vi "line_profile.vi"(0 "Motor COM in":refnum<visa-resource-name>, 1 "Motor error in":errorcluster caption="error out", 2 "Y轴":bool=TRUE, 4 "Keithley COM In":refnum<visa-resource-name>, 5 "Keithley Error In":errorcluster caption="error out", 7 "步长":dbl format="%#_13g", 9 "距离":dbl format="%#_13g", 10 "反向":bool=TRUE) -> (3 "当前位置":dbl format="%#_13g", 12 "XY图":cluster{"X":dbl, "Y":dbl}[](graph), 13 "电流数组":dbl[](array[numeric]), 14 "Motor COM out":refnum<visa-resource-name>, 15 "Motor error out":errorcluster caption="error out", 17 "位移数组":dbl[](array[numeric]), 18 "Keithley COM out":refnum<visa-resource-name>, 19 "Keithley Error out":errorcluster caption="error out")   [LabVIEW 2018]
uses:
  location_x.vi
  location_y.vi
  <instrlib>/Keithley 648X Series/Keithley 648X Series.lvlib
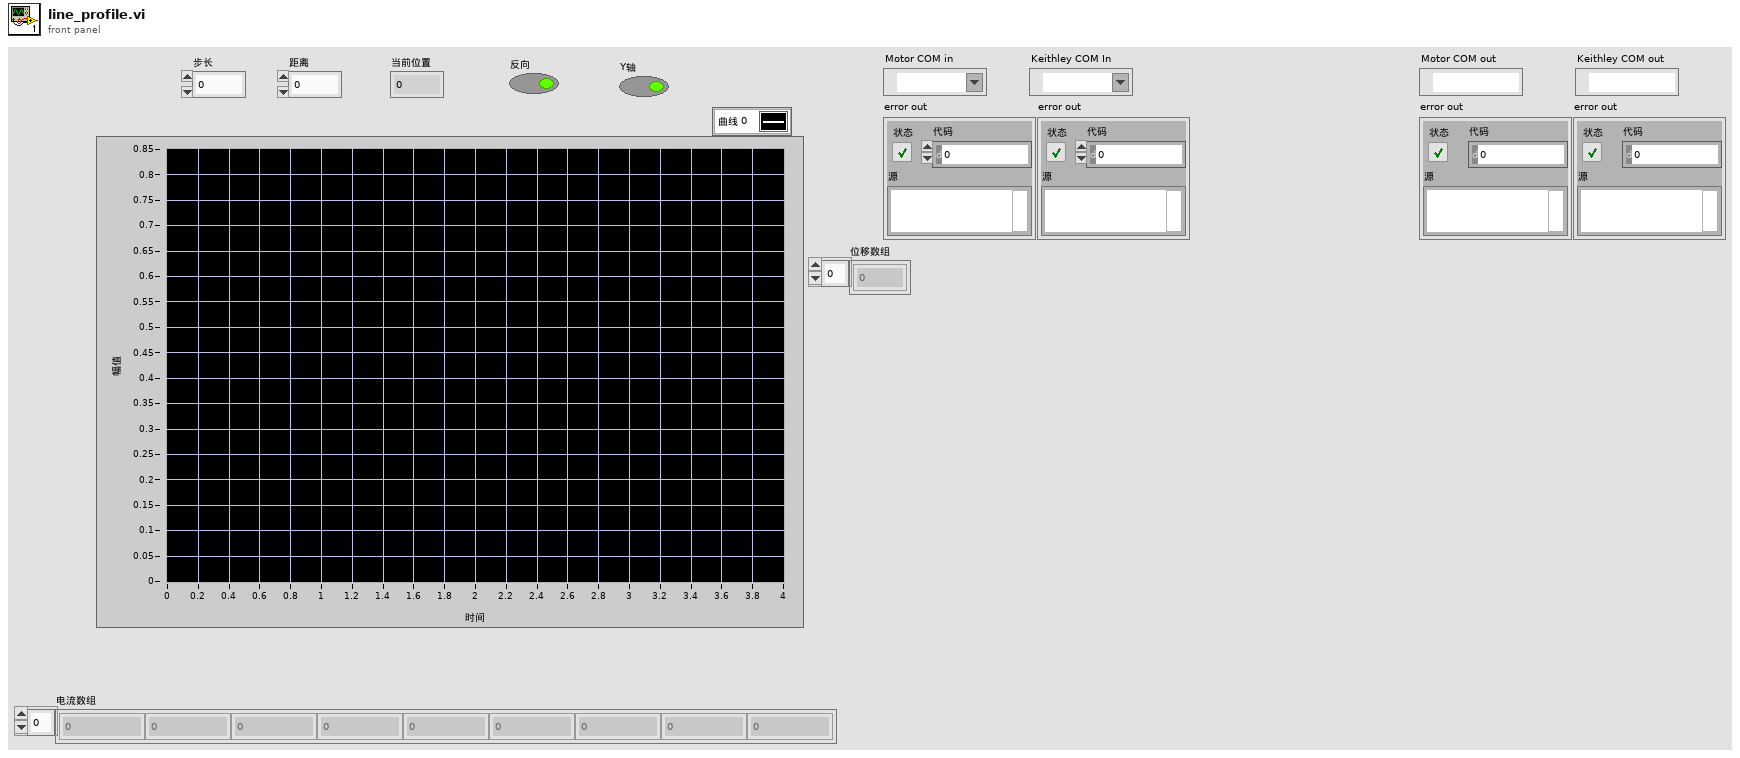
[diagram p1: front panel]
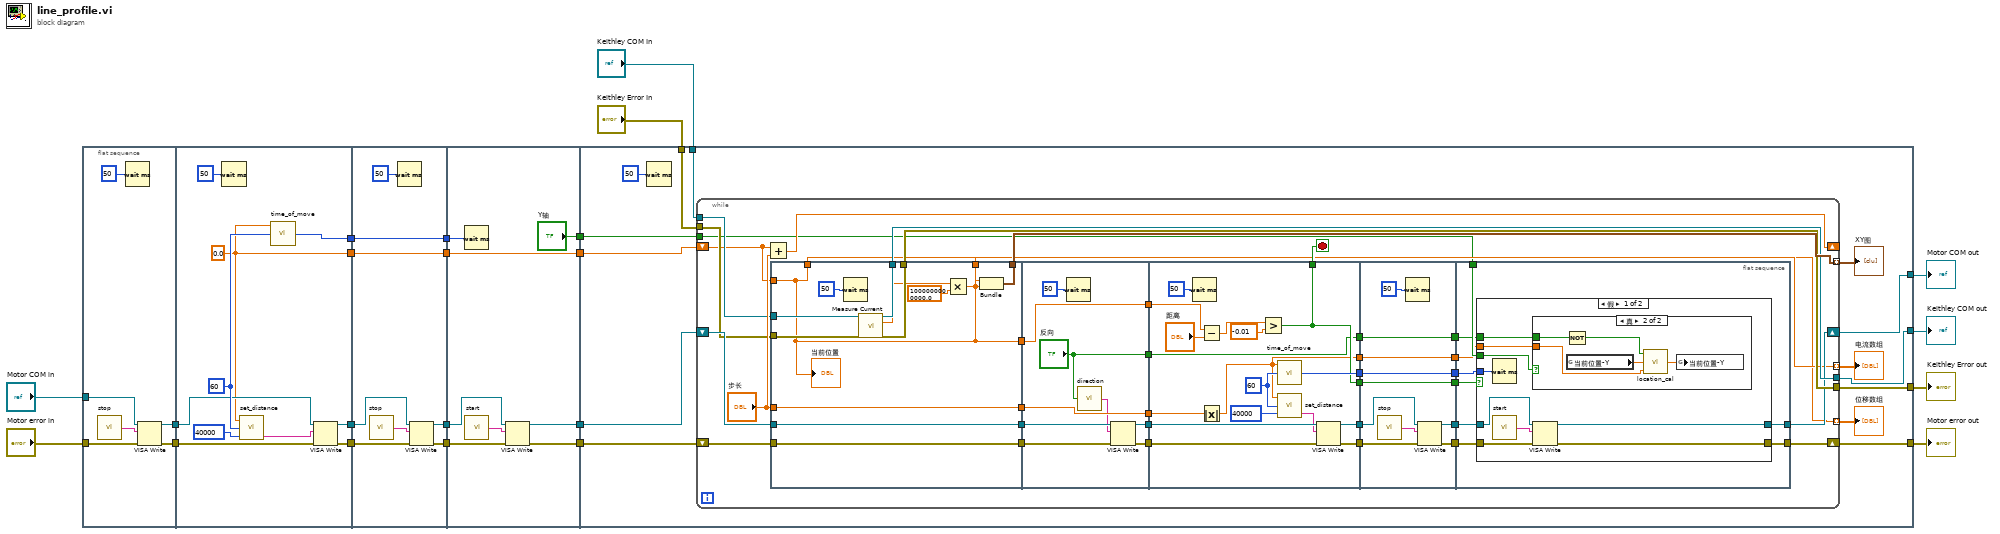
[diagram p0: block diagram]
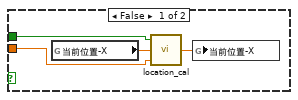
[diagram p2: hidden frame]
diagram:
  n1 = flat-sequence {
    tunnel: "Motor COM in" -> [w28]
    tunnel: "Motor error in" -> [w27]
    tunnel: [w24] -> w22
    tunnel: [w23] -> w21
    tunnel: [w38] -> w20
    tunnel: [w37] -> w19
    tunnel: [w29] -> w18
    tunnel: [w32] -> w17
    tunnel: w22 -> [w31]
    tunnel: w21 -> [w30]
    tunnel: w20 -> [w44]
    tunnel: w19 -> [w46]
    tunnel: [w43] -> w16
    tunnel: [w45] -> w15
    tunnel: [w39] -> w14
    tunnel: w18 -> [w39]
    tunnel: [w40] -> w13
    tunnel: w17 -> [w40]
    tunnel: w16 -> [w52]
    tunnel: w15 -> [w54]
    tunnel: [w51] -> w12
    tunnel: [w53] -> w11
    tunnel: [w49] -> w10
    tunnel: w14 -> [w49]
    tunnel: w13 -> [w48]
    tunnel: ["Y轴"] -> w1
    tunnel: w12 -> [w66]
    tunnel: w11 -> [w68]
    tunnel: w10 -> [w64]
    tunnel: [w65] -> w4
    tunnel: [w67] -> w5
    tunnel: [w59] -> w3
    tunnel: [w58] -> w2
    tunnel: "Keithley Error In" -> [w61]
    tunnel: "Keithley COM In" -> [w60]
    tunnel: w1 -> [w55]
    frame #0 {
      n2 = call "stop.vi"() -> ("指令"=w25:string)
      n3 = Wait (ms)(milliseconds to wait=u32 50 ("毫秒计时值")) -> ()  [unwired: 1 out]
      n4 = VISA Write(VISA resource name=w28, write buffer=w25, error in (no error)=w27) -> (VISA resource name out=w24:refnum<visa-resource-name>, error out=w23:errorcluster)  [unwired: 1 out]
    }
    frame #1 {
      w29 = 0.0
      w33 = i16 60 ("速度(r/min)")
      n5 = Wait (ms)(milliseconds to wait=u32 50 ("毫秒计时值")) -> ()  [unwired: 1 out]
      n6 = call "set_distance.vi"("细分"=40000, "速度(r/min)"=w33, "移动距离(mm)"=w29) -> ("指令"=w35:string)  [unwired: 2 out]
      n7 = call "time_of_move.vi"("转速"=w33, "移动距离"=w29) -> ("所需时间"=w32:i32)  [unwired: 1 in]
      n8 = VISA Write(VISA resource name=w31, write buffer=w35, error in (no error)=w30) -> (VISA resource name out=w37:refnum<visa-resource-name>, error out=w38:errorcluster)  [unwired: 1 out]
    }
    frame #2 {
      n9 = call "stop.vi"() -> ("指令"=w42:string)
      n10 = Wait (ms)(milliseconds to wait=u32 50 ("毫秒计时值")) -> ()  [unwired: 1 out]
      n11 = VISA Write(VISA resource name=w46, write buffer=w42, error in (no error)=w44) -> (VISA resource name out=w45:refnum<visa-resource-name>, error out=w43:errorcluster)  [unwired: 1 out]
    }
    frame #3 {
      n12 = Wait (ms)(milliseconds to wait=w48) -> ()  [unwired: 1 out]
      n13 = call "start.vi"() -> ("指令"=w50:string)
      n14 = VISA Write(VISA resource name=w54, write buffer=w50, error in (no error)=w52) -> (VISA resource name out=w53:refnum<visa-resource-name>, error out=w51:errorcluster)  [unwired: 1 out]
    }
    frame #4 {
      n15 = Wait (ms)(milliseconds to wait=u32 50 ("毫秒计时值")) -> ()  [unwired: 1 out]
      n16 = while {
        shift-right: [w91] -> w67
        shift-left: w68 -> [w105]
        shift-right: [w90] -> w65
        shift-left: w66 -> [w104]
        shift-right: [w88] -> _
        shift-left: w64 -> [w89]
        tunnel: [w94] -> w62 mode=indexing
        tunnel: w61 -> [w95]
        tunnel: w60 -> [w96]
        tunnel: [w93] -> w59
        tunnel: [w92] -> w58
        tunnel: [w76] -> w57 mode=indexing
        tunnel: [w75] -> w56 mode=indexing
        tunnel: w55 -> [w74]
        stop <- w87 stop-if-true
        n17 = Add(x=w89, y="步长") -> (x+y=w88:dbl)
        n18 = flat-sequence {
          tunnel: "步长" -> [w116]
          tunnel: w104 -> [w117]
          tunnel: w105 -> [w118]
          tunnel: [w118] -> w84
          tunnel: [w117] -> w82
          tunnel: [w116] -> w80
          tunnel: w96 -> [w115]
          tunnel: w95 -> [w114]
          tunnel: [w112] -> w94
          tunnel: [w111] -> w93
          tunnel: [w110] -> w92
          tunnel: w89 -> [w108]
          tunnel: [w108] -> w78
          tunnel: [w107] -> w76
          tunnel: [w108] -> w75
          tunnel: w84 -> [w127]
          tunnel: [w124] -> w83
          tunnel: w82 -> [w123]
          tunnel: [w122] -> w81
          tunnel: w80 -> [w125]
          tunnel: [w125] -> w79
          tunnel: w78 -> [w126]
          tunnel: [w126] -> w77
          tunnel: ["反向"] -> w69
          tunnel: [w142] -> w103
          tunnel: [w140] -> w102
          tunnel: [w136] -> w98
          tunnel: w83 -> [w144]
          tunnel: w81 -> [w141]
          tunnel: w79 -> [w135]
          tunnel: [w132] -> w87
          tunnel: w77 -> [w133]
          tunnel: [w132] -> w85
          tunnel: [w129] -> w72
          tunnel: [w128] -> w70
          tunnel: w69 -> [w128]
          tunnel: w103 -> [w153]
          tunnel: w102 -> [w154]
          tunnel: [w152] -> w101
          tunnel: [w151] -> w100
          tunnel: [w148] -> w99
          tunnel: w98 -> [w148]
          tunnel: [w147] -> w86
          tunnel: w85 -> [w147]
          tunnel: [w146] -> w73
          tunnel: w72 -> [w146]
          tunnel: [w145] -> w71
          tunnel: w70 -> [w145]
          tunnel: w101 -> [w163]
          tunnel: w100 -> [w162]
          tunnel: w99 -> [w161]
          tunnel: [w160] -> w91
          tunnel: [w159] -> w90
          tunnel: w86 -> [w158]
          tunnel: w74 -> [w157]
          tunnel: w73 -> [w156]
          tunnel: w71 -> [w155]
          frame #0 {
            n19 = Wait (ms)(milliseconds to wait=u32 50 ("毫秒计时值")) -> ()  [unwired: 1 out]
            n20 = call <instrlib>:"Measure Current.vi"("VISA resource name"=w115, "error in (no error)"=w114) -> ("VISA resource name out"=w111:refnum<visa-resource-name>, "Measurement"=w109:dbl, "error out"=w110:errorcluster)  [unwired: 11 in]
            n21 = Multiply(x=w109, y=1000000000000.0) -> (x*y=w107:dbl)
            n22 = Bundle(w108, w107) -> (w112:cluster{dbl, dbl})  [unwired: 1 in]
            "当前位置" <- w108
          }
          frame #1 {
            n23 = Wait (ms)(milliseconds to wait=u32 50 ("毫秒计时值")) -> ()  [unwired: 1 out]
            n24 = call "direction.vi"("反向"="反向") -> ("指令"=w121:string)
            n25 = VISA Write(VISA resource name=w127, write buffer=w121, error in (no error)=w123) -> (VISA resource name out=w124:refnum<visa-resource-name>, error out=w122:errorcluster)  [unwired: 1 out]
          }
          frame #2 {
            w137 = i16 60 ("速度(r/min)")
            n26 = Wait (ms)(milliseconds to wait=u32 50 ("毫秒计时值")) -> ()  [unwired: 1 out]
            n27 = Subtract(x=w133, y="距离") -> (x-y=w131:dbl)
            n28 = Absolute Value(x=w135) -> (abs(x)=w129:dbl)
            n29 = Greater?(x=w131, y=-0.01) -> (0:w132:bool)
            n30 = call "time_of_move.vi"("转速"=w137, "移动距离"=w129) -> ("所需时间"=w136:i32)  [unwired: 1 in]
            n31 = call "set_distance.vi"("细分"=40000, "速度(r/min)"=w137, "移动距离(mm)"=w129) -> ("指令"=w139:string)  [unwired: 2 out]
            n32 = VISA Write(VISA resource name=w144, write buffer=w139, error in (no error)=w141) -> (VISA resource name out=w142:refnum<visa-resource-name>, error out=w140:errorcluster)  [unwired: 1 out]
          }
          frame #3 {
            n33 = call "stop.vi"() -> ("指令"=w150:string)
            n34 = Wait (ms)(milliseconds to wait=u32 50 ("毫秒计时值")) -> ()  [unwired: 1 out]
            n35 = VISA Write(VISA resource name=w153, write buffer=w150, error in (no error)=w154) -> (VISA resource name out=w152:refnum<visa-resource-name>, error out=w151:errorcluster)  [unwired: 1 out]
          }
          frame #4 {
            n36 = case shown="假" w158 {
              tunnel: w163 -> [w172 w183]
              tunnel: w162 -> [w171 w182]
              tunnel: w161 -> [w169 _]
              tunnel: [w168 w183] -> w160
              tunnel: [w167 w182] -> w159
              tunnel: w157 -> [w166 _]
              tunnel: w156 -> [w165 _]
              tunnel: w155 -> [w164 _]
              frame False {
                n37 = Wait (ms)(milliseconds to wait=w169) -> ()  [unwired: 1 out]
                n38 = call "start.vi"() -> ("指令"=w170:string)
                n39 = case shown="真" w166 {
                  tunnel: w165 -> [w175 w180]
                  tunnel: w164 -> [w173 w178]
                  frame False {
                    n40 = global read "location_x.vi" "当前位置-X"() -> (w176:dbl)
                    n41 = call "location_cal.vi"("移动距离"=w175, "当前位置"=w176, "反向"=w173) -> ("结束位置"=w174:dbl)
                    n42 = global write "location_x.vi" "当前位置-X"(w174) -> ()
                  }
                  frame True {
                    n43 = Not(x=w178) -> (.not. x?=w177:bool)
                    n44 = global read "location_y.vi" "当前位置-Y"() -> (w181:dbl)
                    n45 = call "location_cal.vi"("移动距离"=w180, "当前位置"=w181, "反向"=w177) -> ("结束位置"=w179:dbl)
                    n46 = global write "location_y.vi" "当前位置-Y"(w179) -> ()
                  }
                }
                n47 = VISA Write(VISA resource name=w172, write buffer=w170, error in (no error)=w171) -> (VISA resource name out=w168:refnum<visa-resource-name>, error out=w167:errorcluster)  [unwired: 1 out]
              }
              frame True {
              }
            }
          }
        }
      }
      "XY图" <- w62
      "电流数组" <- w57
      "位移数组" <- w56
    }
  }
  "Motor COM out" <- w5
  "Motor error out" <- w4
  "Keithley COM out" <- w3
  "Keithley Error out" <- w2
